vi "Connect to Slave.vi"(8 "error in (no error)":errorcluster, 11 "TEST in":refnum<class "TEST.lvclass">) -> (0 "error out":errorcluster, 3 "TEST out":refnum<class "TEST.lvclass">)   [LabVIEW 2021, in "TEST.lvclass"]
uses:
  TEST.lvclass
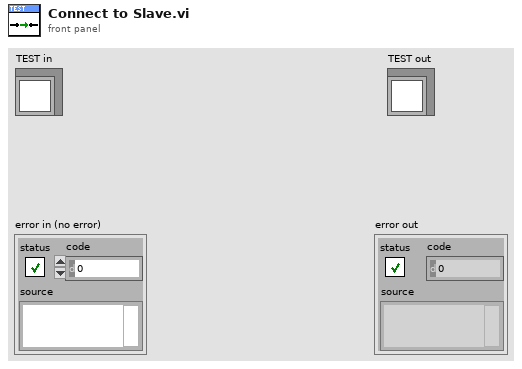
[diagram p1: front panel]
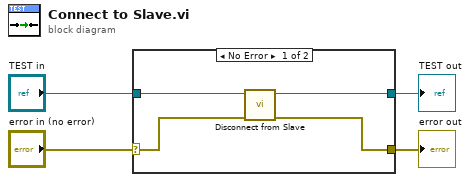
[diagram p0: block diagram]
diagram:
  n1 = case shown="No Error" "error in (no error)" {
    selector: "error in (no error)" -> [w7 w9]
    tunnel: [w5 w9] -> w3
    tunnel: [w6 w10] -> w4
    tunnel: "TEST in" -> [w8 w10]
    frame No Error {
      n2 = call-dynamic "Disconnect from Slave.vi"("error in"=w7, "TCP master in"=w8) -> ("error out"=w5:errorcluster, "TCP master out"=w6:refnum<class "TEST.lvclass">)  [unwired: 8 in]
    }
    frame Error {
    }
  }
  "error out" <- w3
  "TEST out" <- w4
